vi "Close.vi"(8 "error in":errorcluster, 11 "Limit in":refnum<class "Limit.lvclass">) -> (0 "error out":errorcluster, 3 "Limit out":refnum<class "Limit.lvclass">)   [LabVIEW 2023, in "Limit.lvclass"]
uses:
  Limit.lvclass
  Limit.lvclass/Limit.ctl
  <vilib>/ADAS Replay HIL/AdasHilServices/AdasHilServices Fill In Error Info Ex.vi
  <vilib>/ADAS Replay HIL/AdasHilServices/AdasHilChannelServices.lvlib
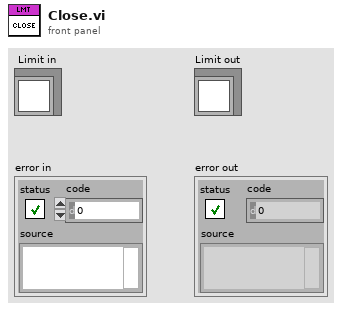
[diagram p1: front panel]
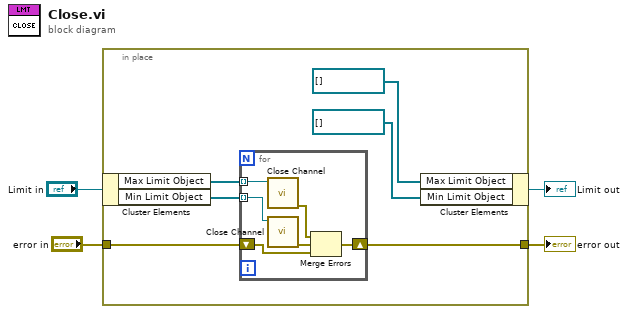
[diagram p0: block diagram]
diagram:
  n1 = in-place {
    in-place-border: "error in" -> [w10]
    in-place-border: [w9] -> w2
    n2 = in-place-cluster #1("Limit in") -> ("Max Limit Object"=w8:refnum<k21>[], "Min Limit Object"=w7:refnum<k21>[])
    n3 = for {
      tunnel: w8 -> [w16] mode=indexing
      tunnel: w7 -> [w15] mode=indexing
      shift-right: [w14] -> w9
      shift-left: w10 -> [w11]
      n4 = call <vilib>:"Close Channel.vi"("ADAS HIL Channel"=w16) -> ("error out"=w13:errorcluster)  [unwired: 10 in]
      n5 = call <vilib>:"Close Channel.vi"("ADAS HIL Channel"=w15) -> ("error out"=w12:errorcluster)  [unwired: 10 in]
      n6 = Merge Errors(w13, w12, w11) -> (w14:errorcluster)
    }
    n7 = in-place-cluster #1("Max Limit Object"=refnum<k21>[] [] ("Control Mode Read"), "Min Limit Object"=refnum<k21>[] [] ("Control Mode Read")) -> (→"Limit out":refnum<class "Limit.lvclass">)
  }
  "error out" <- w2
